vi "Reserve FPGA Resource.vi"(7 "notes":string, 8 "error in (no error)":errorcluster, 9 "Name in Bitfile":string, 10 "Server Ref in":T1 format="%.0x", 11 "Item Ref in":T1 format="%.0x") -> (0 "error out":errorcluster, 3 "Item Ref out":T1 format="%.0x")   [LabVIEW 2016, in "FPGA RM System Definition API.lvlib"]
uses:
  System Definition/FPGA RM System Definition API.lvlib
  <vilib>/NI Veristand/Custom Device API/Custom Device Item Ref.ctl
  <vilib>/NI VeriStand/Custom Device API/Custom Device API.lvlib
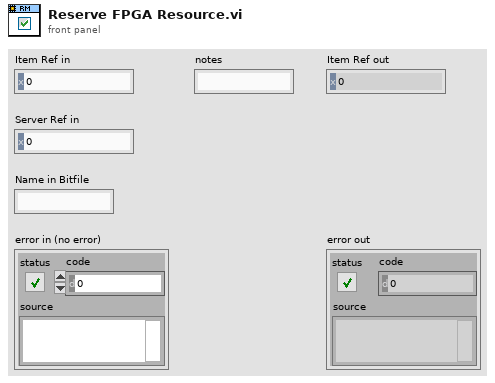
[diagram p1: front panel]
types:
  T1 = typedef "Custom Device API.lvlib/Custom Device Item Ref.ctl" = u64
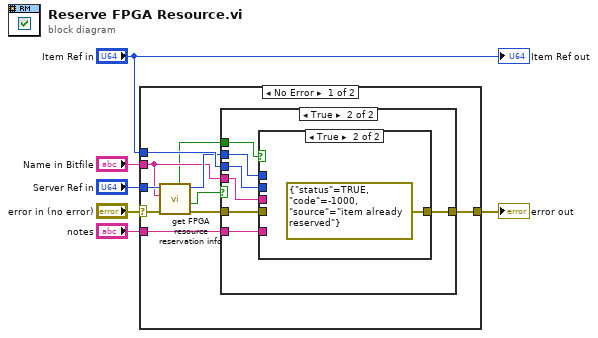
[diagram p0: block diagram]
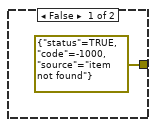
[diagram p2: hidden frame]
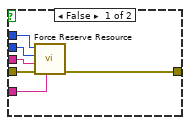
[diagram p3: hidden frame]
diagram:
  n1 = case shown="No Error" "error in (no error)" {
    selector: "error in (no error)" -> [w9 w32]
    tunnel: [w14 w32] -> w5
    tunnel: "Item Ref in" -> [w15 _]
    tunnel: "Server Ref in" -> [w13 _]
    tunnel: "notes" -> [w16 _]
    tunnel: "Name in Bitfile" -> [w11 _]
    frame No Error {
      n2 = call "get FPGA resource reservation info.vi"("error in (no error)"=w9, "Name in Bitfile"=w11, "Item Ref in"=w13) -> ("error out"=w8:errorcluster, "found?"=w10:bool, "Item Ref out"=w12:T1, "reserved?"=w7:bool)  [unwired: 3 in, 2 out]
      n3 = case shown="True" w10 {
        tunnel: w16 -> [_ w19]
        tunnel: w15 -> [_ w24]
        tunnel: w8 -> [_ w23]
        tunnel: [errorcluster {"status"=TRUE, "code"=-1000, "source"="item not found"} ("error out") w22] -> w14
        tunnel: w12 -> [_ w21]
        tunnel: w11 -> [_ w20]
        tunnel: w7 -> [_ w18]
        frame False {
        }
        frame True {
          n4 = case shown="True" w18 {
            tunnel: w24 -> [w30 _]
            tunnel: w23 -> [w29 _]
            tunnel: [w28 errorcluster {"status"=TRUE, "code"=-1000, "source"="item already reserved"} ("error out")] -> w22
            tunnel: w21 -> [w27 _]
            tunnel: w20 -> [w26 _]
            tunnel: w19 -> [w25 _]
            frame False {
              n5 = call "Force Reserve Resource.vi"("notes"=w25, "error in (no error)"=w29, "Name in bitfile"=w26, "Client Node Ref"=w30, "Item Ref in"=w27) -> ("error out"=w28:errorcluster)  [unwired: 5 in, 1 out]
            }
            frame True {
            }
          }
        }
      }
    }
    frame Error {
    }
  }
  "error out" <- w5
  "Item Ref out" <- "Item Ref in"
